vi "test 3- NonCSMCallsWorkerMode_UseAPI.vi"(8 "error in (no error)":errorcluster, 11 "TestCase in":refnum<class "testcase-SyncMessage.lvclass">) -> (0 "error out":errorcluster, 3 "TestCase out":refnum<class "testcase-SyncMessage.lvclass">)   [LabVIEW 2017, in "testcase-SyncMessage.lvclass"]
uses:
  testcase-SyncMessage.lvclass
  _support/SyncMessage_CSM_Callee.vi
  <vilib>/addons/_JKI Toolkits/VI Tester/TestCase.llb/TestCase.lvclass
  src/user.lib/_NEVSTOP/Communicable State Machine(CSM)/Communicable State Machine.lvlib
  C:/Program Files (x86)/National Instruments/LabVIEW 2017/vi.lib/addons/_JKI Toolkits/VI Tester/TestCase.llb/TestCase.lvclass
panel:
  out ">> Msg/Rep's CSM >>":string
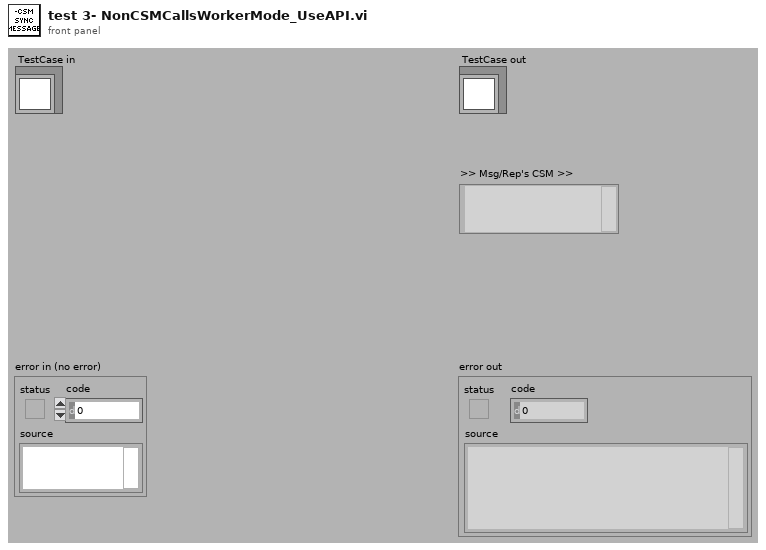
[diagram p1: front panel]
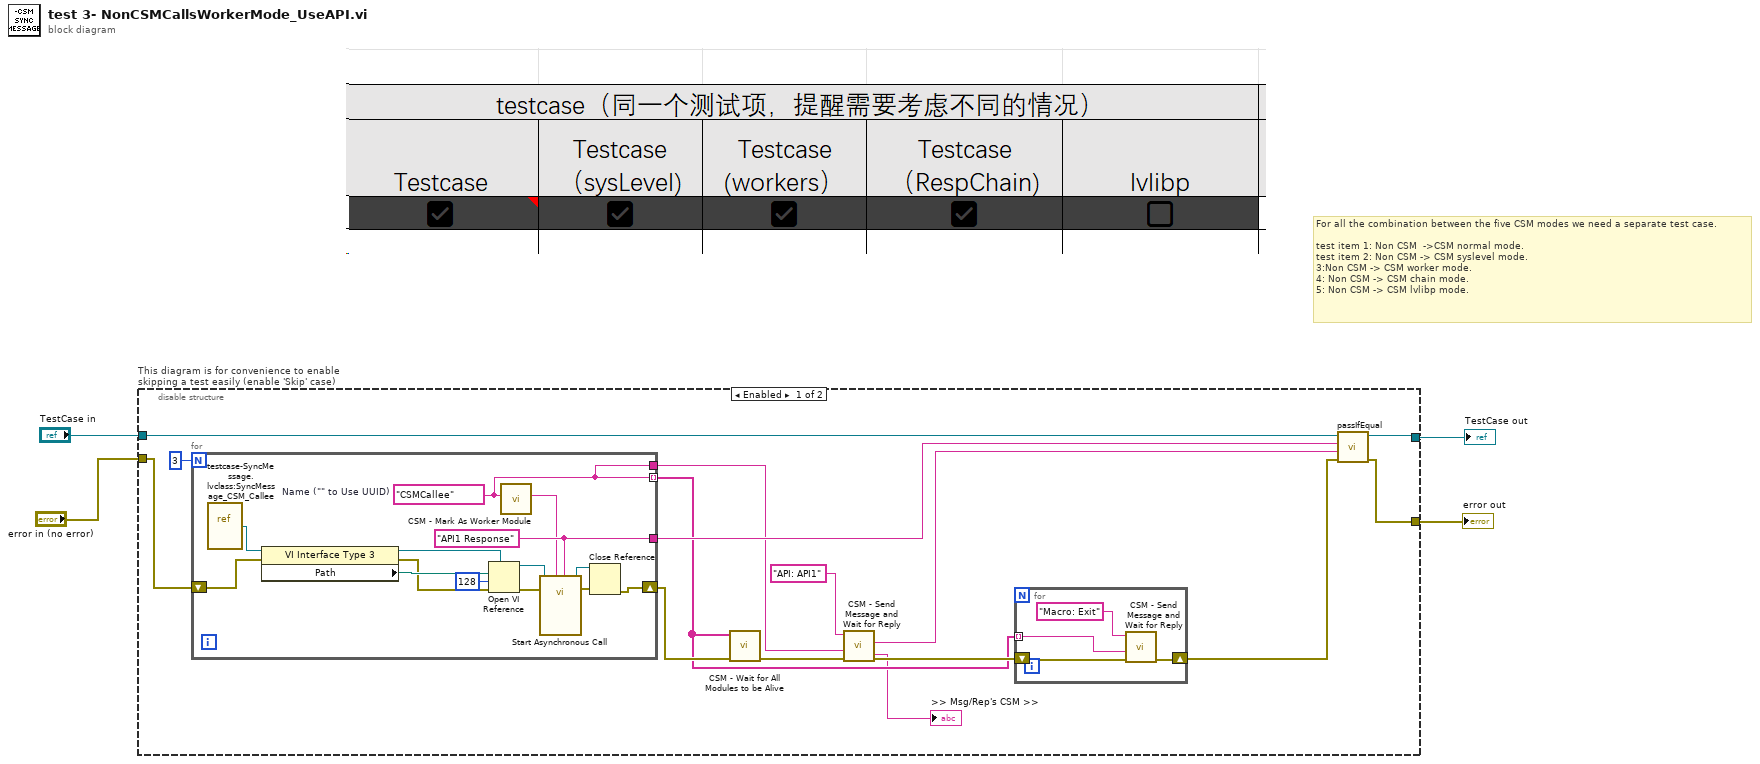
[diagram p0: block diagram]
diagram:
  # "For all the combination between the five CSM modes we need a separate test case.\n\ntest item 1: Non CSM  ->CSM normal mode.\ntest item 2: Non CSM -> CSM syslevel mode.\n3:Non CSM -> CSM worker mode.\n4: Non CSM -> CSM chain mode.\n5: Non CSM -> CSM lvlibp mode."
  n1 = disable-structure "This diagram is for convenience to enable skipping a test easily (enable 'Skip' case)" shown="Enabled" {
    disable-tunnel: "TestCase in" -> [w19 w41]
    disable-tunnel: [w18 w39] -> w2
    disable-tunnel: [w17 w40] -> w1
    disable-tunnel: "error in (no error)" -> [w11 w38]
    frame Enabled {
      n2 = for {
        N: 3 -> [_]
        tunnel: [w23] -> w10
        shift-right: [w22] -> w8
        shift-left: w11 -> [w24]
        tunnel: [w21] -> w6 mode=indexing
        tunnel: [w21] -> w7
        w23 = "API1 Response" ("API response in")
        w21 = "CSMCallee"  # Name ("" to Use UUID)
        n3 = vi-ref "testcase-SyncMessage.lvclass:SyncMessage_CSM_Callee.vi"() -> (w32:refnum<vi>)
        n4 = property class="VI Interface Type 3"(reference=w32, error in=w24) -> (reference out=w28:refnum<vi>, error out=w30:errorcluster, "Path"=w31:path)
        n5 = Open VI Reference(type specifier VI Refnum (for type only)=w28, vi path=w31, options=128, error in (no error)=w30) -> (vi reference=w29:refnum<vi>, error out=w33:errorcluster)  [unwired: 2 in]
        n6 = call "CSM - Mark As Worker Module.vi"("CSM Name"=w21) -> ("CSM Name (Marked As Worker)"=w20:string)  [unwired: 9 in]
        n7 = call-by-ref "Start Asynchronous Call"(reference=w29, error in=w33, "API response in"=w23, "Name (\"\" to Use UUID)"=w20) -> (reference out=w26:refnum<vi>, error out=w27:errorcluster)  [unwired: 10 in]
        n8 = Close Reference(reference=w26, error in (no error)=w27) -> (error out=w22:errorcluster)
      }
      n9 = call "CSM - Wait for All Modules to be Alive.vi"("Error In"=w8, "CSM Names"=w6) -> ("error out"=w15:errorcluster)  [unwired: 7 in, 2 out]
      n10 = call "CSM - Send Message and Wait for Reply.vi"("Error In (No Error)"=w15, "Target Module"=w7, "State"="API: API1") -> ("error out"=w12:errorcluster, "Response"=w13:string, ">> Msg/Rep's CSM >>"=→">> Msg/Rep's CSM >>":string)  [unwired: 6 in]
      n11 = for {
        shift-right: [w36] -> w16
        shift-left: w12 -> [w37]
        tunnel: w6 -> [w34] mode=indexing
        n12 = call "CSM - Send Message and Wait for Reply.vi"("Error In (No Error)"=w37, "Target Module"=w34, "State"="Macro: Exit") -> ("error out"=w36:errorcluster)  [unwired: 6 in, 2 out]
      }
      n13 = call-dynamic "passIfEqual.vi"("error in (no error)"=w16, "y"=w13, "x"=w10, "TestCase in"=w19) -> ("error out"=w17:errorcluster, "TestCase out"=w18:refnum<class "testcase-SyncMessage.lvclass">)  [unwired: 6 in]
    }
    frame Disabled {
      # "skip test result while test is under development"
      n14 = call <vilib>:"skip.vi"("error in (no error)"=w38, "TestCase in"=w41) -> ("error out"=w40:errorcluster, "TestCase out"=w39:refnum<class "testcase-SyncMessage.lvclass">)  [unwired: 8 in]
    }
  }
  "error out" <- w1
  "TestCase out" <- w2
